vi "Queue.vi"(4 "Enum":T1, 8 "error in (no error)":errorcluster, 10 "Enqueue Element":string) -> (0 "error out":errorcluster, 1 "remaining elements":string[](array[string]), 2 "Dequeued Element":string)   [LabVIEW 2020]
uses:
  Typedef/QueueOperation.ctl
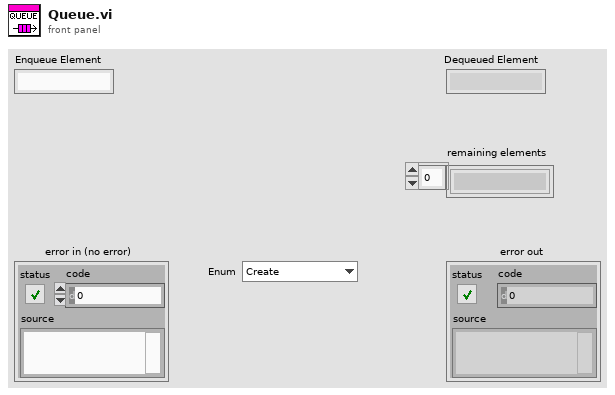
[diagram p1: front panel]
types:
  T1 = typedef "QueueOperation.ctl" = enum16{"Create", "Enqueue", "Dequeue", "Flush", "Close"}
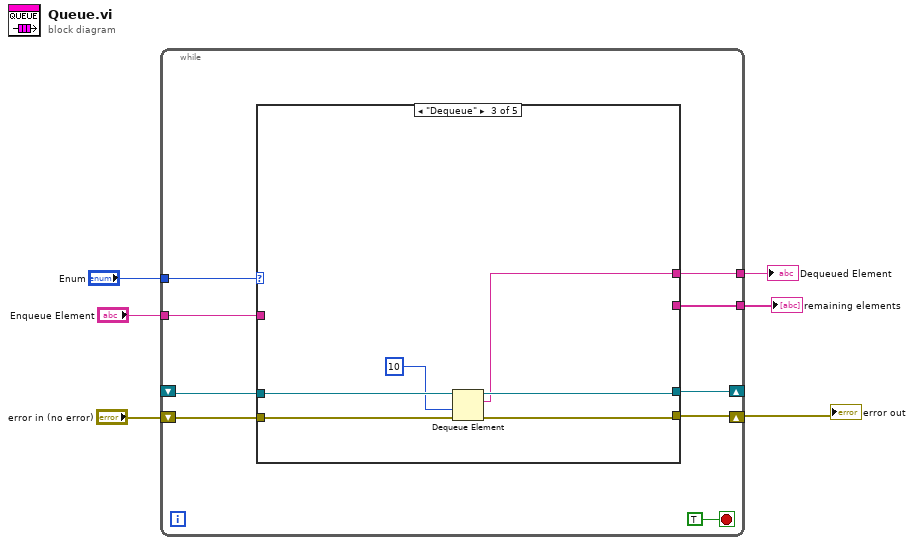
[diagram p0: block diagram]
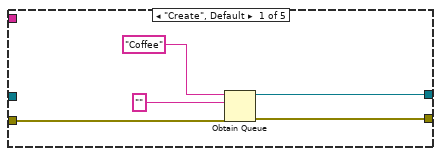
[diagram p2: hidden frame]
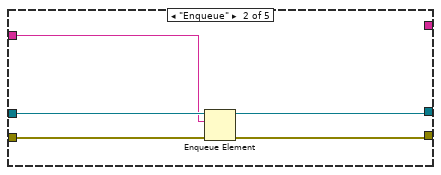
[diagram p3: hidden frame]
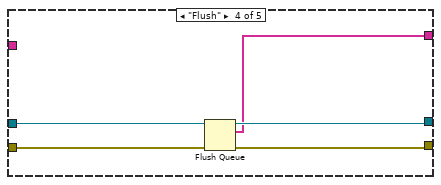
[diagram p4: hidden frame]
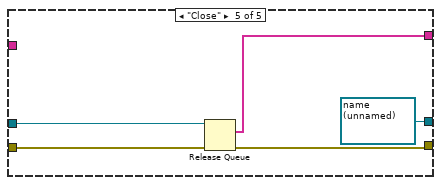
[diagram p5: hidden frame]
diagram:
  n1 = while {
    tunnel: "Enum" -> [w14]
    shift-right: [w12] -> w4
    shift-left: "error in (no error)" -> [w13]
    shift-right: [w11] -> _
    shift-left: _ -> [w10]
    tunnel: "Enqueue Element" -> [w9]
    tunnel: [w8] -> w2
    tunnel: [w7] -> w1
    stop <- TRUE stop-if-true
    n2 = case shown="\"Dequeue\"" w14 {
      tunnel: w13 -> [w20 w25 w31 w36 w41]
      tunnel: [w19 w24 w30 w35 w40] -> w12
      tunnel: [w16 w23 w28 w33 refnum<queue> refnum ("queue out")] -> w11
      tunnel: w10 -> [_ w22 w29 w34 w39]
      tunnel: w9 -> [_ w21 _ _ _]
      tunnel: [_ _ _ w32 w37] -> w8
      tunnel: [_ _ w26 _ _] -> w7
      frame "Create", Default {
        n3 = Obtain Queue(name (unnamed)="Coffee", element data type="" ("name (unnamed)"), error in (no error)=w20) -> (queue out=w16:refnum<queue>, error out=w19:errorcluster)  [unwired: 2 in, 1 out]
      }
      frame "Enqueue" {
        n4 = Enqueue Element(queue=w22, element=w21, error in (no error)=w25) -> (queue out=w23:refnum<queue>, error out=w24:errorcluster)  [unwired: 1 in, 1 out]
      }
      frame "Dequeue" {
        n5 = Dequeue Element(queue=w29, timeout in ms (-1)=10, error in (no error)=w31) -> (queue out=w28:refnum<queue>, element=w26:string, error out=w30:errorcluster)  [unwired: 1 out]
      }
      frame "Flush" {
        n6 = Flush Queue(queue=w34, error in (no error)=w36) -> (queue out=w33:refnum<queue>, remaining elements=w32:string[], error out=w35:errorcluster)
      }
      frame "Close" {
        n7 = Release Queue(queue=w39, error in (no error)=w41) -> (remaining elements=w37:string[], error out=w40:errorcluster)  [unwired: 1 in, 1 out]
      }
    }
  }
  "error out" <- w4
  "remaining elements" <- w2
  "Dequeued Element" <- w1
